vi "写D+12字符+文本.vi"(8 "error out":errorcluster, 9 "文本输入":string, 10 "输入地址D":i32, 11 "VISA resource name out":refnum<visa-resource-name>) -> (0 "error out 2":errorcluster caption="error out", 2 "通讯延时":u32, 3 "VISA resource name out 2":refnum<visa-resource-name>, 4 "连接的字符串":string, 5 "读取缓冲区":string)   [LabVIEW 2012]
uses:
  <vilib>/Instr/_visa.llb/VISA Configure Serial Port (Instr).vi
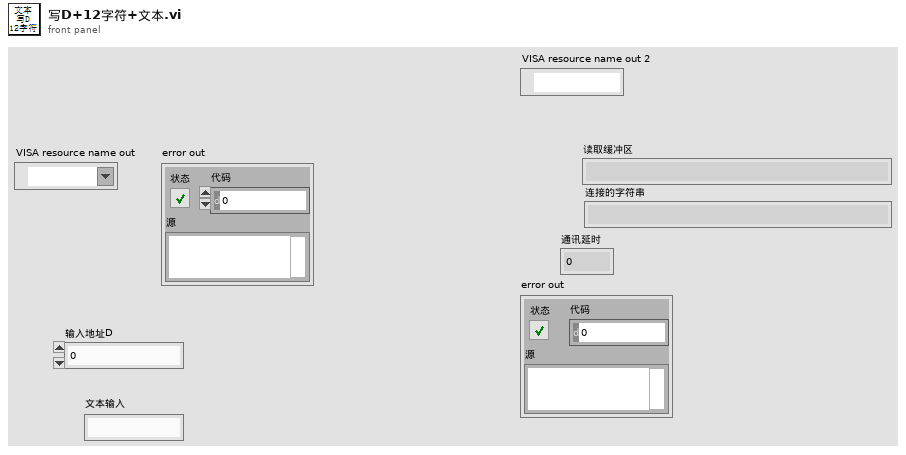
[diagram p1: front panel]
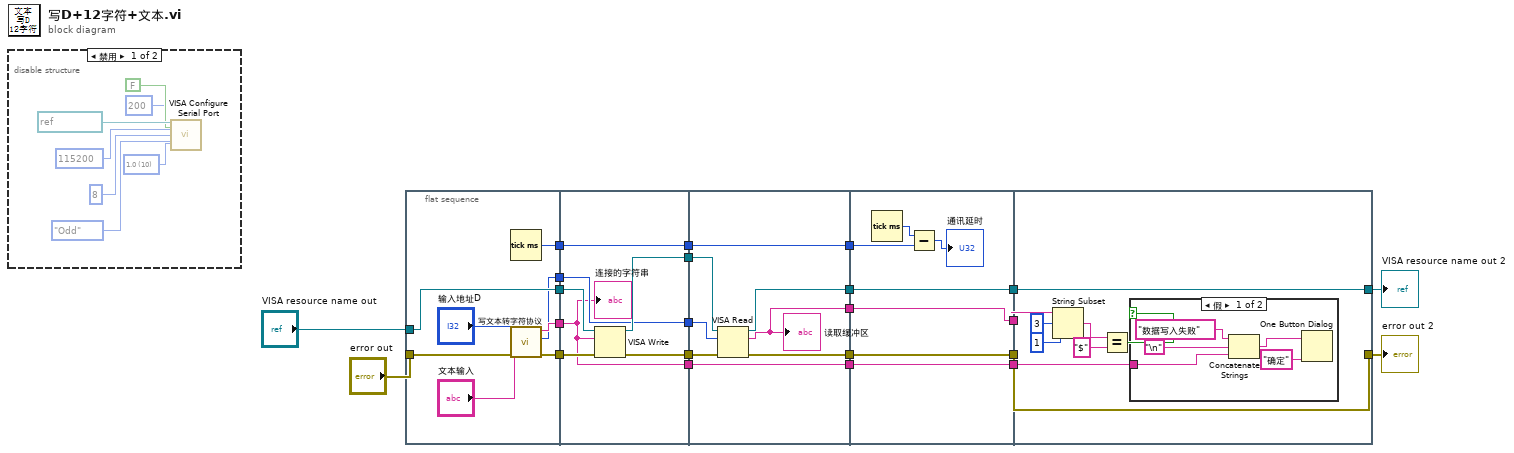
[diagram p0: block diagram]
diagram:
  n1 = disable-structure shown="禁用" {
    frame Disabled {
      w26 = u16 10 items=["1.0"=10, "1.5"=15, "2.0"=20] ("stop bits (10: 1 bit)")
      n2 = call-poly "VISA Configure Serial Port"("VISA resource name"=refnum<visa-resource-name> "COM3", "timeout (10sec)"=u32 200, "Enable Termination\nChar (T)"=FALSE ("Enable Termination\nChar (T)"), "baud rate (9600)"=u32 115200, "data bits (8)"=u16 8, "parity (0:none)"=enum16{"None", "Odd", "Even", "Mark", "Space"}."Odd", "stop bits (10: 1 bit)"=w26) -> ()  [unwired: 7 in, 2 out]
    }
    frame Enabled {
    }
  }
  n3 = flat-sequence {
    tunnel: "VISA resource name out" -> [w37]
    tunnel: "error out" -> [w36]
    tunnel: [w37] -> w23
    tunnel: [w36] -> w22
    tunnel: [w35] -> w21
    tunnel: [w34] -> w17
    tunnel: [w33] -> w16
    tunnel: w23 -> [w43]
    tunnel: w22 -> [w44]
    tunnel: w21 -> [w38]
    tunnel: [w42] -> w20
    tunnel: [w41] -> w19
    tunnel: [w40] -> w18
    tunnel: w17 -> [w40]
    tunnel: w16 -> [w39]
    tunnel: [w39] -> w15
    tunnel: [w38] -> w1
    tunnel: w20 -> [w50]
    tunnel: w19 -> [w49]
    tunnel: w18 -> [w48]
    tunnel: w15 -> [w47]
    tunnel: [w52] -> w14
    tunnel: [w51] -> w13
    tunnel: [w47] -> w12
    tunnel: [w46] -> w8
    tunnel: [w45] -> w2
    tunnel: w1 -> [w45]
    tunnel: w14 -> [w59]
    tunnel: w13 -> [w58]
    tunnel: w12 -> [w56]
    tunnel: [w59] -> w11
    tunnel: [w58] -> w10
    tunnel: [w54] -> w9
    tunnel: w8 -> [w54]
    tunnel: [w53] -> w3
    tunnel: w2 -> [w53]
    tunnel: [w67] -> w4
    tunnel: [w68] -> w5
    tunnel: w11 -> [w68]
    tunnel: w10 -> [w67]
    tunnel: w9 -> [w66]
    tunnel: w3 -> [w60]
    frame #0 {
      n4 = Tick Count (ms)() -> (millisecond timer value=w33:u32)
      n5 = call "写文本转字符协议.vi"("输入文本"="文本输入", "输入地址"="输入地址D") -> ("返回字节数"=w34:u16, "连接的字符串"=w35:string)  [unwired: 8 in]
    }
    frame #1 {
      n6 = VISA Write(VISA resource name=w43, write buffer=w38, error in (no error)=w44) -> (VISA resource name out=w42:refnum<visa-resource-name>, error out=w41:errorcluster)  [unwired: 1 out]
      "连接的字符串" <- w38
    }
    frame #2 {
      n7 = VISA Read(VISA resource name=w50, byte count=w48, error in (no error)=w49) -> (VISA resource name out=w52:refnum<visa-resource-name>, read buffer=w46:string, error out=w51:errorcluster)  [unwired: 1 out]
      "读取缓冲区" <- w46
    }
    frame #3 {
      n8 = Tick Count (ms)() -> (millisecond timer value=w57:u32)
      n9 = Subtract(x=w57, y=w56) -> (x-y=→"通讯延时":u32)
    }
    frame #4 {
      n10 = String Subset(string=w66, offset (0)=3 ("偏移量(0)"), length (rest)=1 ("长度（剩余）")) -> (substring=w63:string)
      n11 = Equal?(x=w63, y="$") -> (x = y?=w61:bool)
      n12 = case shown="假" w61 {
        tunnel: w60 -> [w70 _]
        frame False {
          n13 = Concatenate Strings("数据写入失败" ("消息"), "\n", w70) -> (w69:string)
          n14 = One Button Dialog(message=w69, button name ("OK")="确定" ("按钮名称（“确定”）")) -> ()  [unwired: 1 out]
        }
        frame True {
        }
      }
    }
  }
  "VISA resource name out 2" <- w5
  "error out 2" <- w4
